vi "p05.vi"() -> ()   [LabVIEW 2019]
uses:
  Control 1.ctl
  <vilib>/Platform/TimedLoop/XDataNode/timing_clust.ctl
  <vilib>/Platform/TimedLoop/XDataNode/nitl_modes.ctl
  <vilib>/Platform/TimedLoop/XDataNode/wakeup.ctl
  <vilib>/DAQmx/read.llb/DAQmx Read (Analog 1D DBL 1Chan NSamp).vi
  <vilib>/Analysis/baseanly.llb/Mean (DBL).vi
  <vilib>/DAQmx/create/channels.llb/DAQmx Create Channel (AI-Voltage-Basic).vi
  <vilib>/DAQmx/configure/timing.llb/DAQmx Timing (Sample Clock).vi
  <vilib>/DAQmx/miscellaneous.llb/DAQmx Fill In Error Info.vi
  <vilib>/Utility/file.llb/Write Delimited Spreadsheet (DBL).vi
  <vilib>/platform/TimedLoop/XDataNode/XDataNode.xnode
  <vilib>/Platform/TimedLoop/XDataNode/XDNodeRunTimeDep.lvlib
  <vilib>/Analysis/NI_AALBase.lvlib
panel:
  in  "Cantidad de Muestras":i32
  in  "Cantidad de mediciones por muestra":i32
  in  "Tiempo de espera":i32
  out "Tiempo":string
  out "Estado Actual":string
  in  "Valor T0":dbl=298.15
  in  "Valor Beta":dbl=4100.0
  in  "Valor Resistencia":dbl=10000.0
  in  "Inicio":bool
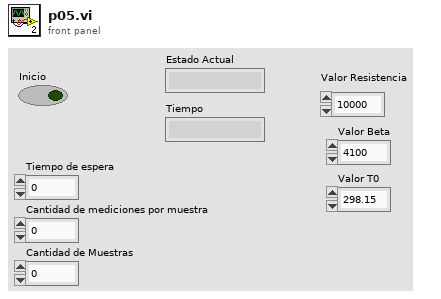
[diagram p1: front panel]
types:
  T1 = typedef "Control 1.ctl" = enum16{"stand-by", "medida", "espera", "final"}
  T2 = typedef "XDNodeRunTimeDep.lvlib/timing_clust.ctl" = cluster{"Expected End [f-1]":u64, "Actual End [f-1]":u64, "Finished Late? [f-1]":bool, "Expected End [i-1]":u64, "Actual End [i-1]":u64, "Finished Late? [i-1]":bool, "Expected Start [i]":u64, "Actual Start [i]":u64, "Expected Start [f]":u64, "Actual Start [f]":u64, "Source Name":string, "Structure Name":string, "Period":i64, "Deadline":i64, "Offset":i64, "Start":i64, "Priority":i32, "Timeout":i32, "Mode":T3, "Wakeup Reason":T4, "Error":errorcluster, "Source Type":string, "Secondary Source Type":string, "Global End Time":u64, "Global Start Time":u64, "Frame Duration":u64, "Iteration Duration":u64, "Assigned CPU":i32, "I/O Scan Engine Mode":u32}
  T3 = typedef "XDNodeRunTimeDep.lvlib/nitl_modes.ctl" = enum32{"No Change", "Process missed periods, maintain original phase", "Discard missed periods, maintain original phase", "Process missed periods, ignore original phase", "Discard missed periods, ignore original phase"}
  T4 = typedef "XDNodeRunTimeDep.lvlib/wakeup.ctl" = enum32{"Normal", "Aborted", "Asynchronous wakeup", "Timing source error", "Timed loop error", "Timeout"}
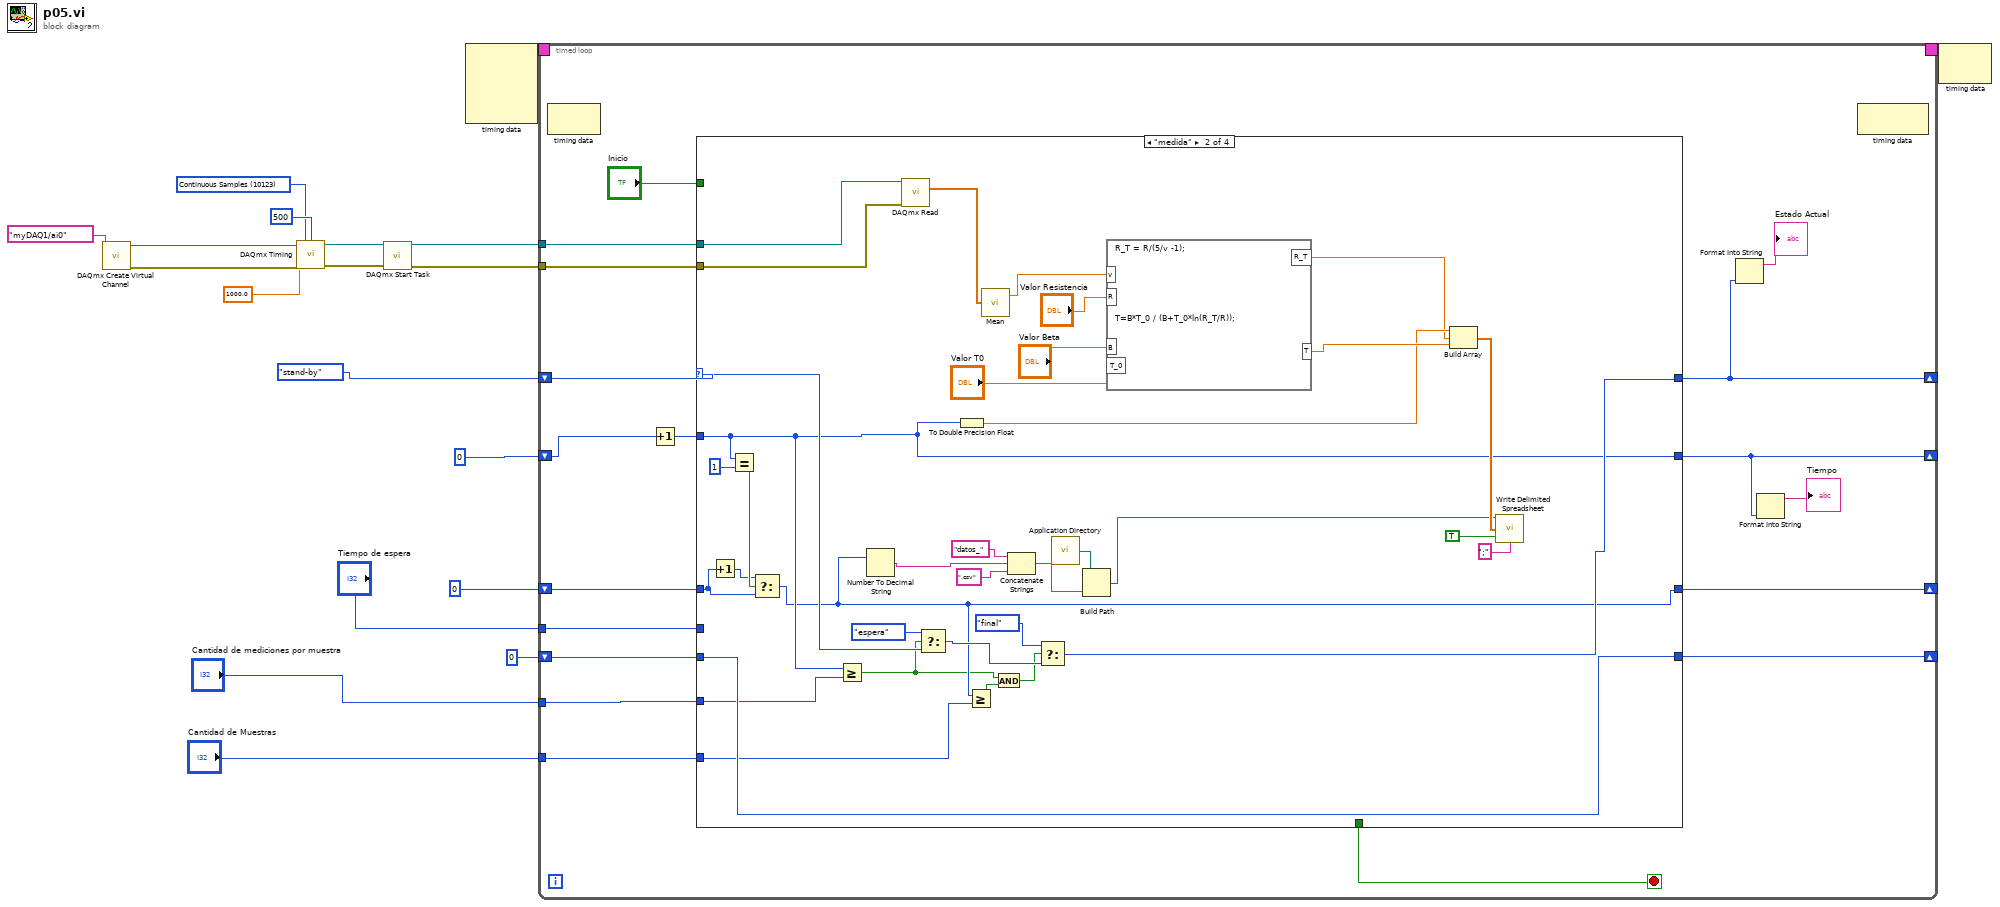
[diagram p0: block diagram]
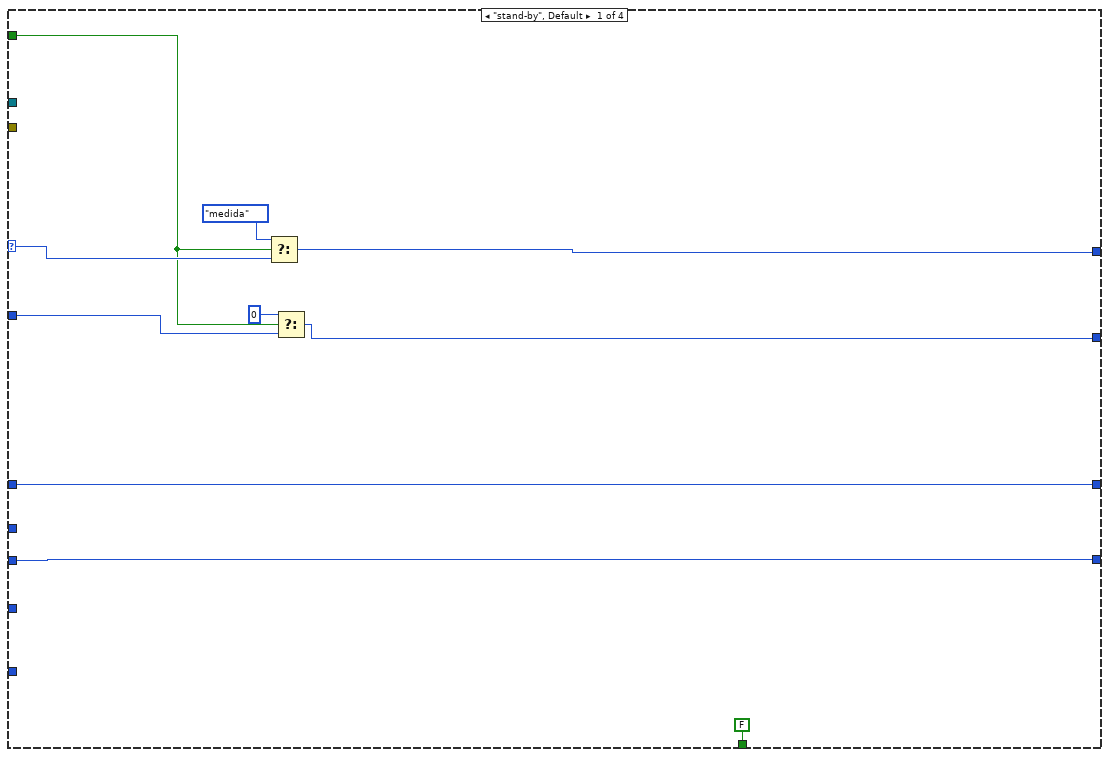
[diagram p2: hidden frame]
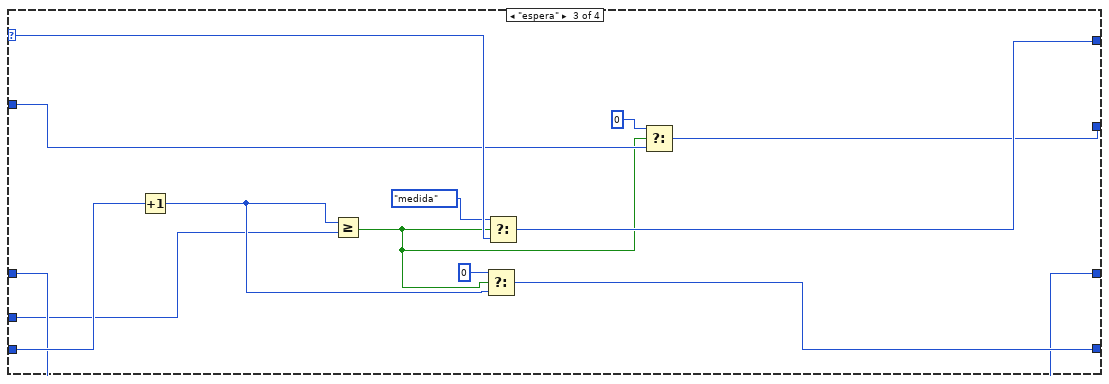
[diagram p3: hidden frame]
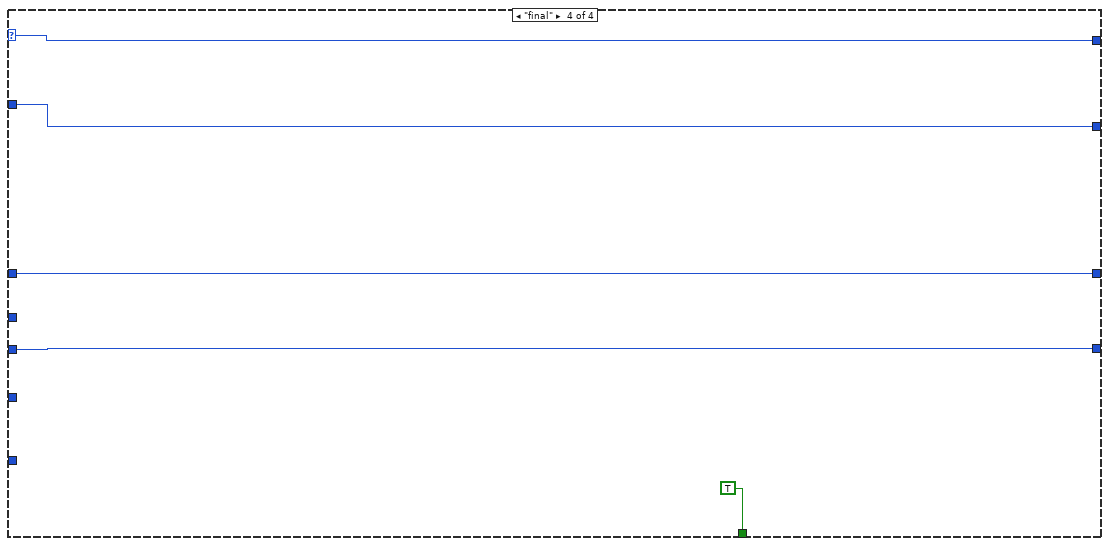
[diagram p4: hidden frame]
diagram:
  w13 = 10123 items=["Finite Samples"=10178, "Continuous Samples"=10123, "Hardware Timed Single Point"=12522] ("sample mode")
  n1 = call-poly <vilib>:"DAQmx Create Virtual Channel.vi"("physical channels"=tag "myDAQ1/ai0") -> ("task out"=w19:refnum<k21>, "error out"=w18:errorcluster)  [unwired: 13 in]
  n2 = call-poly <vilib>:"DAQmx Timing.vi"("task/channels in"=w19, "sample mode"=w13, "samples per channel"=500, "rate"=1000.0, "error in"=w18) -> ("task out"=w15:refnum<k21>, "error out"=w14:errorcluster)  [unwired: 9 in]
  n3 = call <vilib>:"DAQmx Start Task.vi"("task/channels in"=w15, "error in"=w14) -> ("task out"=w9:refnum<k21>, "error out"=w8:errorcluster)  [unwired: 12 in]
  n4 = node-c288() -> (w11:T2)  [unwired: 4 in]
  n5 = timed-loop {
    timing: w11 -> [_]
    timing-out: [_] -> w10
    tunnel: w9 -> [w37]
    tunnel: w8 -> [w36]
    shift-right: [w28] -> _
    shift-left: Control_1."stand-by" -> [w35]
    shift-right: [w23] -> _
    shift-left: 0 -> [w32]
    shift-right: [w29] -> _
    shift-left: 0 -> [w30]
    shift-right: [w25] -> _
    shift-left: 0 -> [w26]
    tunnel: "Tiempo de espera" -> [w22]
    tunnel: "Cantidad de mediciones por muestra" -> [w21]
    tunnel: "Cantidad de Muestras" -> [w20]
    stop <- w33 stop-if-true
    n6 = node-c288() -> ()  [unwired: 1 in, 1 out]
    n7 = Increment(x=w32) -> (x+1=w31:i32)
    n8 = case shown="\"medida\"" w35 {
      selector: w35 -> [w47 w64 w95 w100]
      tunnel: w37 -> [_ w83 _ _]
      tunnel: w36 -> [_ w82 _ _]
      tunnel: "Inicio" -> [w42 _ _ _]
      tunnel: [w45 w61 w93 w100] -> w28
      tunnel: w31 -> [w43 w54 w88 w99]
      tunnel: [w40 w54 w87 w99] -> w23
      tunnel: [FALSE _ _ TRUE] -> w33
      tunnel: w30 -> [w39 w59 w96 w98]
      tunnel: [w39 w59 w90 w98] -> w29
      tunnel: w26 -> [w38 w52 w85 w97]
      tunnel: [w38 w51 w85 w97] -> w25
      tunnel: w22 -> [_ _ w84 _]
      tunnel: w21 -> [_ w55 _ _]
      tunnel: w20 -> [_ w53 _ _]
      frame "stand-by", Default {
        n9 = Select(t=Control_1."medida", s=w42, f=w47) -> (s? t:f=w45:T1)
        n10 = Select(t=0, s=w42, f=w43) -> (s? t:f=w40:i32)
      }
      frame "medida" {
        n11 = Increment(x=w52) -> (x+1=w56:i32)
        n12 = Equal?(x=w54, y=1) -> (x = y?=w57:bool)
        n13 = Select(t=w56, s=w57, f=w52) -> (s? t:f=w51:i32)
        n14 = Greater Or Equal?(x=w54, y=w55) -> (x >= y?=w48:bool)
        n15 = Number To Decimal String(number=w51) -> (decimal integer string=w65:string)  [unwired: 1 in]
        n16 = call-poly <vilib>:"DAQmx Read.vi"("task/channels in"=w83, "error in"=w82) -> ("data"=w77:dbl[])  [unwired: 11 in, 2 out]
        n17 = Select(t=Control_1."espera", s=w48, f=w64) -> (s? t:f=w62:T1)
        n18 = To Double Precision Float(number=w54) -> (double precision float=w75:dbl)
        n19 = Greater Or Equal?(x=w51, y=w53) -> (x >= y?=w49:bool)
        n20 = call-poly <vilib>:"Mean.vi"("X"=w77) -> ("mean"=w81:dbl)  [unwired: 1 out]
        n21 = And(x=w48, y=w49) -> (x .and. y?=w50:bool)
        n22 = Concatenate Strings("datos_" ("string"), w65, ".csv" ("string")) -> (w68:string)
        n23 = Select(t=Control_1."final", s=w50, f=w62) -> (s? t:f=w61:T1)
        n24 = call <vilib>:"Application Directory.vi"() -> ("Application Directory"=w70:path)
        n25 = Build Path(base path=w70, name or relative path=w68) -> (appended path=w66:path)
        n26 = formula code="R_T = R/(5/v -1);\n\n\n\n\n\n\nT=B*T_0 / (B+T_0*ln(R_T/R));"("v"=w81, "B"="Valor Beta", "T_0"="Valor T0", "R"="Valor Resistencia") -> ("R_T"=w74:dbl, "T"=w76:dbl)
        n27 = Build Array(w75, w74, w76) -> (w71:dbl[])
        n28 = call-poly <vilib>:"Write Delimited Spreadsheet.vi"("file path (dialog if empty)"=w66, "1D data"=w71, "append to file? (new file:F)"=TRUE, "delimiter (\\t)"=";" ("delimiter (\\t)")) -> ()  [unwired: 10 in, 2 out]
      }
      frame "espera" {
        n29 = Increment(x=w96) -> (x+1=w91:i32)
        n30 = Greater Or Equal?(x=w91, y=w84) -> (x >= y?=w86:bool)
        n31 = Select(t=0, s=w86, f=w91) -> (s? t:f=w90:i32)
        n32 = Select(t=Control_1."medida", s=w86, f=w95) -> (s? t:f=w93:T1)
        n33 = Select(t=0, s=w86, f=w88) -> (s? t:f=w87:i32)
      }
      frame "final" {
      }
    }
    n34 = Format Into String(w28) -> (resulting string=→"Estado Actual":string)  [unwired: 3 in, 1 out]
    n35 = Format Into String(w23) -> (resulting string=→"Tiempo":string)  [unwired: 3 in, 1 out]
    n36 = node-c288() -> ()  [unwired: 1 in, 1 out]
  }
  n37 = node-c288(w10) -> ()  [unwired: 1 out]
